vi "HumanTrajPositions.vi"(10 "FieldPos":T1(ring), 11 "Init":bool) -> (1 "vAngular":dbl, 2 "vY":dbl, 3 "vX":dbl)   [LabVIEW 2023]
uses:
  <vilib>/Rock Robotics/WPI/ThirdParty/JAS_Junk/TrajLib/Trajectory_Library.lvlib
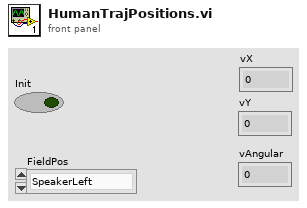
[diagram p1: front panel]
types:
  T1 = enum16{"SpeakerLeft", "SpeakerCenter", "SpeakerRight", "Amp", "Source", "StageLeft", "StageCenter", "StageRight"}
  T2 = typedef "WPI_DriverStationAllianceInfo.ctl" = enum16{"Red", "Blue", "Invalid"}
  T3 = typedef "Trajectory_Library.lvlib/POSE2D.ctl" = cluster{"TRANSLATION":T4, "ROTATION":T5}
  T4 = typedef "Trajectory_Library.lvlib/TRANSLATION2D.ctl" = cluster{"X":dbl, "Y":dbl}
  T5 = typedef "Trajectory_Library.lvlib/ROTATION2D.ctl" = cluster{"VALUE":dbl, "COS":dbl, "SIN":dbl}
  T6 = typedef "Trajectory_Library.lvlib/CHASSIS_SPEEDS.ctl" = cluster{"vX":dbl, "vY":dbl, "vOmega":dbl}
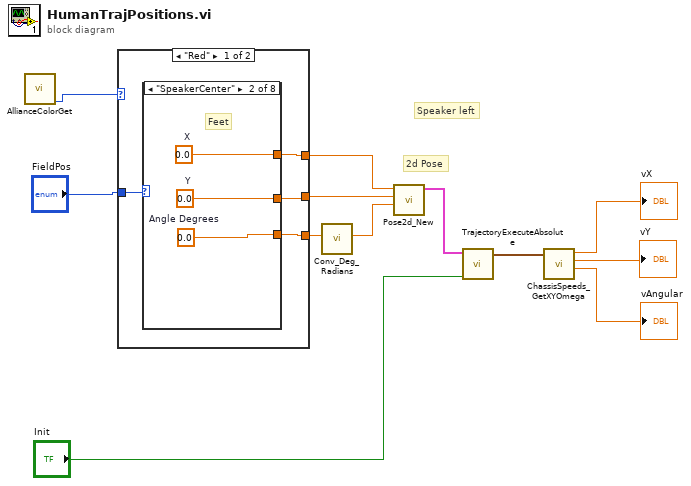
[diagram p0: block diagram]
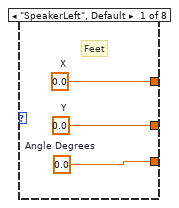
[diagram p2: hidden frame]
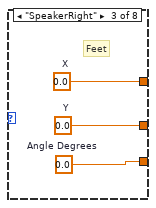
[diagram p3: hidden frame]
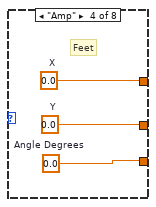
[diagram p4: hidden frame]
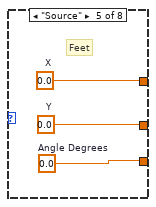
[diagram p5: hidden frame]
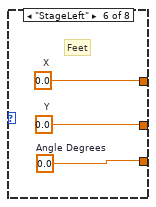
[diagram p6: hidden frame]
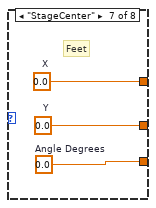
[diagram p7: hidden frame]
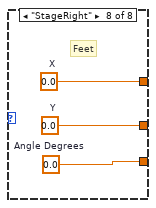
[diagram p8: hidden frame]
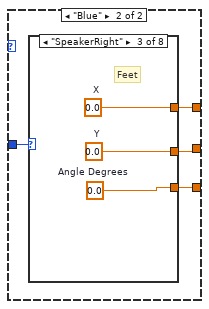
[diagram p9: hidden frame]
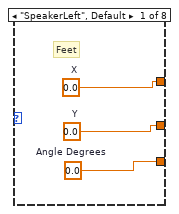
[diagram p10: hidden frame]
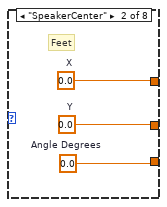
[diagram p11: hidden frame]
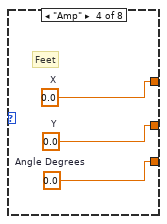
[diagram p12: hidden frame]
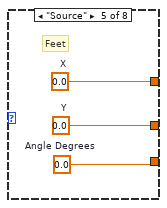
[diagram p13: hidden frame]
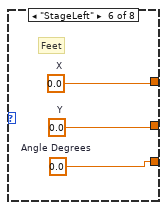
[diagram p14: hidden frame]
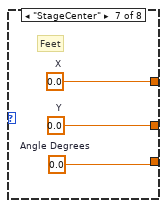
[diagram p15: hidden frame]
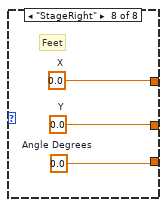
[diagram p16: hidden frame]
diagram:
  # "2d Pose"
  # "Speaker left"
  n1 = call "AllianceColorGet.vi"() -> ("AllianceColor"=w1:T2)  [unwired: 11 in]
  n2 = case shown="\"Red\"" w1 {
    tunnel: [w14 w44] -> w11
    tunnel: [w15 w43] -> w9
    tunnel: [w16 w42] -> w8
    tunnel: "FieldPos" -> [w13 w41]
    frame "Red" {
      n3 = case shown="\"SpeakerCenter\"" w13 {
        tunnel: [w17 w20 w25 w26 w29 w32 w35 w40] -> w14
        tunnel: [w18 w21 w24 w27 w30 w33 w36 w39] -> w15
        tunnel: [w19 w22 w23 w28 w31 w34 w37 w38] -> w16
        frame "SpeakerLeft", Default {
          w19 = 0.0  # X
          w18 = 0.0  # Y
          w17 = 0.0  # Angle Degrees
          # "Feet"
        }
        frame "SpeakerCenter" {
          w22 = 0.0  # X
          w21 = 0.0  # Y
          w20 = 0.0  # Angle Degrees
          # "Feet"
        }
        frame "SpeakerRight" {
          w23 = 0.0  # X
          w24 = 0.0  # Y
          w25 = 0.0  # Angle Degrees
          # "Feet"
        }
        frame "Amp" {
          w28 = 0.0  # X
          w27 = 0.0  # Y
          w26 = 0.0  # Angle Degrees
          # "Feet"
        }
        frame "Source" {
          w31 = 0.0  # X
          w30 = 0.0  # Y
          w29 = 0.0  # Angle Degrees
          # "Feet"
        }
        frame "StageLeft" {
          w34 = 0.0  # X
          w33 = 0.0  # Y
          w32 = 0.0  # Angle Degrees
          # "Feet"
        }
        frame "StageCenter" {
          w37 = 0.0  # X
          w36 = 0.0  # Y
          w35 = 0.0  # Angle Degrees
          # "Feet"
        }
        frame "StageRight" {
          w38 = 0.0  # X
          w39 = 0.0  # Y
          w40 = 0.0  # Angle Degrees
          # "Feet"
        }
      }
    }
    frame "Blue" {
      n4 = case shown="\"SpeakerRight\"" w41 {
        tunnel: [w45 w48 w53 w54 w57 w60 w63 w66] -> w44
        tunnel: [w46 w49 w52 w55 w58 w61 w64 w67] -> w43
        tunnel: [w47 w50 w51 w56 w59 w62 w65 w68] -> w42
        frame "SpeakerLeft", Default {
          w47 = 0.0  # X
          w46 = 0.0  # Y
          w45 = 0.0  # Angle Degrees
          # "Feet"
        }
        frame "SpeakerCenter" {
          w50 = 0.0  # X
          w49 = 0.0  # Y
          w48 = 0.0  # Angle Degrees
          # "Feet"
        }
        frame "SpeakerRight" {
          w51 = 0.0  # X
          w52 = 0.0  # Y
          w53 = 0.0  # Angle Degrees
          # "Feet"
        }
        frame "Amp" {
          w56 = 0.0  # X
          w55 = 0.0  # Y
          w54 = 0.0  # Angle Degrees
          # "Feet"
        }
        frame "Source" {
          w59 = 0.0  # X
          w58 = 0.0  # Y
          w57 = 0.0  # Angle Degrees
          # "Feet"
        }
        frame "StageLeft" {
          w62 = 0.0  # X
          w61 = 0.0  # Y
          w60 = 0.0  # Angle Degrees
          # "Feet"
        }
        frame "StageCenter" {
          w65 = 0.0  # X
          w64 = 0.0  # Y
          w63 = 0.0  # Angle Degrees
          # "Feet"
        }
        frame "StageRight" {
          w68 = 0.0  # X
          w67 = 0.0  # Y
          w66 = 0.0  # Angle Degrees
          # "Feet"
        }
      }
    }
  }
  n5 = call <vilib>:"Conv_Deg_Radians.vi"("Degress"=w11) -> ("Radians"=w10:dbl)  [unwired: 10 in]
  n6 = call <vilib>:"Pose2d_New.vi"("Heading"=w10, "Y"=w9, "X"=w8) -> ("out POSe"=w12:T3)  [unwired: 8 in]
  n7 = call "TrajectoryExecuteAbsolute.vi"("Init"="Init", "End Pose ENG"=w12) -> ("Chassis Velocity Target"=w7:T6)  [unwired: 8 in, 1 out]
  n8 = call <vilib>:"ChassisSpeeds_GetXYOmega.vi"("CHASSIS"=w7) -> ("vAngular"=→"vAngular":dbl, "vY"=→"vY":dbl, "vX"=→"vX":dbl)  [unwired: 8 in]
